vi "a.vi"() -> ()   [LabVIEW 2013]
uses:
  controls/Data.ctl
panel:
  out "error out":errorcluster
  in  "error in (no error)":errorcluster
  out "Data":T1
  # "日期"
  # "機種名稱"
  # "機種代號"
  # "商品條碼"
  # "OK"
  # "台"
  # "NG"
  # "總計"
  # "台"
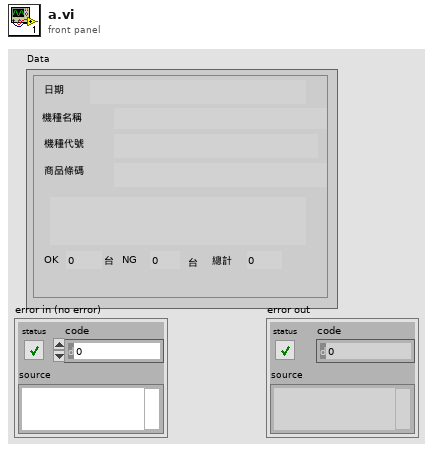
[diagram p1: front panel]
types:
  T1 = typedef "Data.ctl" = cluster{"Date":string, "BarCode1":string, "BarCode2":string, "BarCode3":string, "Message":string, "OK Count":u16, "NG Count":u16, "Total Count":u16, "ModelData":string[][], "OK&NG":bool, "COM1":refnum<visa-resource-name>, "COM2":refnum<visa-resource-name>, "IO":i32, "Time":u32}
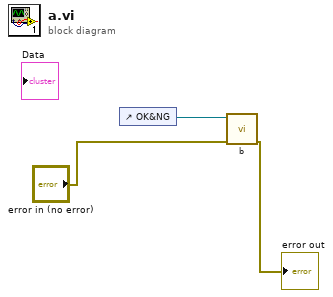
[diagram p0: block diagram]
diagram:
  n1 = control-ref of="OK&NG"() -> (w3:refnum<vi>)
  n2 = call "b.vi"("error in (no error)"="error in (no error)", "OK&NG"=w3) -> ("error out"=→"error out":errorcluster)  [unwired: 8 in, 1 out]
